vi "Packetize.vi"(8 "Error In":errorcluster, 9 "ARGS":u8[](array[numeric]), 10 "CMD":u16, 11 "LINX Device Config":T1) -> (0 "Error Out":errorcluster, 2 "Packet":string, 3 "LINX Decice Config":T1)   [LabVIEW 2013, in "LVH-LINX.lvlib" / "Device.lvlib"]
doc: "This VI takes a LINX command and arguments and builds a LINX packet."
uses:
  <vilib>/LabVIEW Hacker/LINX/Private/Device/Device.lvlib
  <vilib>/LabVIEW Hacker/LINX/Private/Device/Type Defs/LINX Device Config.ctl
  <vilib>/LabVIEW Hacker/LINX/Private/Type Defs/Interface.ctl
  <vilib>/LabVIEW Hacker/LINX/Private/Device/Type Defs/TCP Config.ctl
  <vilib>/LabVIEW Hacker/LINX/Private/Type Defs/Device Family.ctl
  <vilib>/LabVIEW Hacker/LINX/Private/Device/Type Defs/Packet Number FGV Action.ctl
  <vilib>/LabVIEW Hacker/LINX/LVH-LINX.lvlib
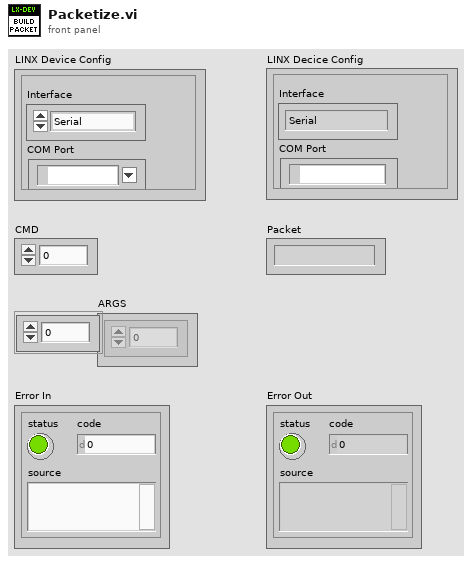
[diagram p1: front panel]
types:
  T1 = typedef "LVH-LINX.lvlib/Device.lvlib/LINX Device Config.ctl" = cluster{"Interface":T2, "COM Port":refnum<visa-resource-name>, "TCP Configuration":T3, "Device Family":T4, "Device ID":u8, "Device Name":string, "TCP Ref":refnum<k5>}
  T2 = typedef "LVH-LINX.lvlib/Interface.ctl" = enum16{"Serial", "TCP"}
  T3 = typedef "LVH-LINX.lvlib/Device.lvlib/TCP Config.ctl" = cluster{"IP Address":string, "Port":u16}
  T4 = typedef "LVH-LINX.lvlib/Device Family.ctl" = enum8{"National Instruments", "Digilent", "Arduino"}
  T5 = typedef "LVH-LINX.lvlib/Device.lvlib/Packet Number FGV Action.ctl" = enum16{"Initialize", "Get", "Increment"}
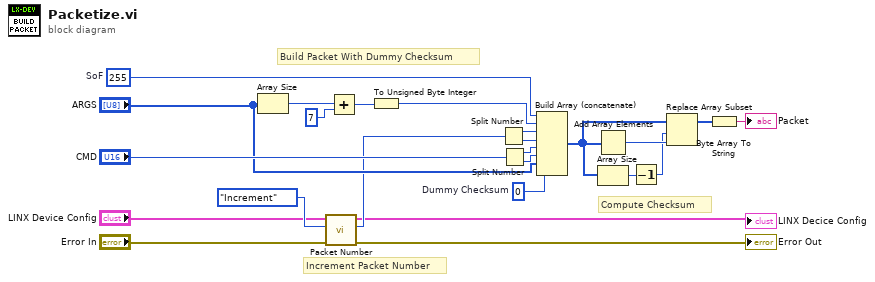
[diagram p0: block diagram]
diagram:
  w13 = u8 0  # Dummy Checksum
  w22 = u8 255  # SoF
  # "Increment Packet Number"
  # "Build Packet With Dummy Checksum"
  # "Compute Checksum"
  n1 = Array Size(array="ARGS") -> (size(s)=w24:i32)
  n2 = call <vilib>:"Packet Number.vi"("Error In"="Error In", "Action"=Packet_Number_FGV_Action."Increment", "LINX Device Config"="LINX Device Config") -> ("Error Out"=→"Error Out":errorcluster, "Packet Number"=w3:u16, "LINX Device Config"=→"LINX Decice Config":T1)  [unwired: 6 in]
  n3 = Add(x=w24, y=7) -> (x+y=w21:i32)
  n4 = To Unsigned Byte Integer(number=w21) -> (unsigned 8bit integer=w20:u8)
  n5 = Split Number(x=w3) -> (hi(x)=w19:u8, lo(x)=w18:u8)
  n6 = Split Number(x="CMD") -> (hi(x)=w17:u8, lo(x)=w16:u8)
  n7 = Build Array (concatenate)(w22, w20, w19, w18, w17, w16, "ARGS", w13) -> (w12:u8[])
  n8 = Add Array Elements(numeric array=w12) -> (sum=w11:u8)
  n9 = Array Size(array=w12) -> (size(s)=w8:i32)
  n10 = Decrement(x=w8) -> (x-1=w7:i32)
  n11 = Replace Array Subset(array=w12, new element=w11, index=w7) -> (w10:u8[])
  n12 = Byte Array To String(unsigned byte array=w10) -> (string=→"Packet":string)
